vi "Write object configuration.vi"(4 "Present":bool=TRUE, 6 "Object name":string, 8 "Error In":errorcluster, 9 "Configuration":variant, 10 "File path":path, 11 "object":refnum<class>) -> (0 "Error Out":errorcluster, 1 "Section out":string, 2 "File path out":path)   [LabVIEW 2019]
uses:
  <vilib>/Utility/config.llb/NI_LVConfig.lvlib
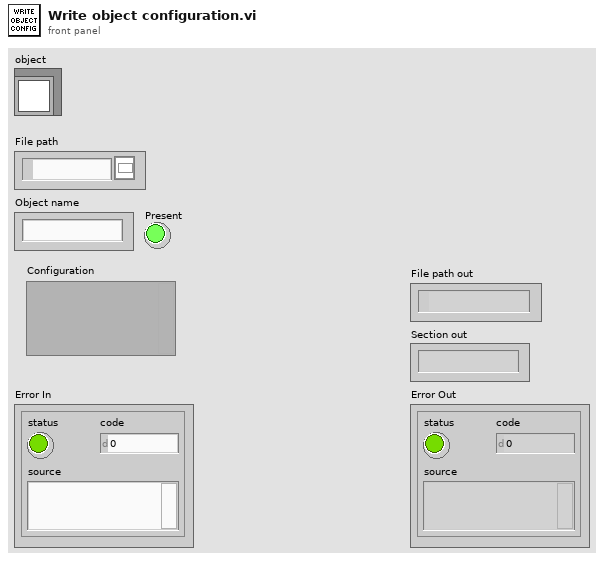
[diagram p1: front panel]
types:
  T1 = typedef "NI_LVConfig.lvlib/Config Data RefNum.ctl" = refnum<k1>
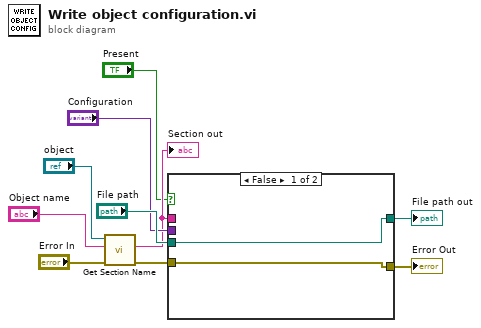
[diagram p0: block diagram]
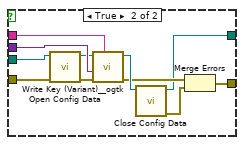
[diagram p2: hidden frame]
diagram:
  n1 = call "Get Section Name.vi"("Error In"="Error In", "Object name"="Object name", "object"="object") -> ("Error Out"=w3:errorcluster, "Section out"=w4:string)  [unwired: 7 in]
  "Section out" <- w4
  n2 = case shown="False" "Present" {
    tunnel: "File path" -> [w12 w23]
    tunnel: "Configuration" -> [_ w22]
    tunnel: [w12 w16] -> w8
    tunnel: [w11 w15] -> w7
    tunnel: w4 -> [_ w14]
    tunnel: w3 -> [w11 w13]
    frame False {
    }
    frame True {
      n3 = call <vilib>:"Open Config Data.vi"("error in (no error)"=w13, "configuration file path"=w23) -> ("error out"=w20:errorcluster, "refnum"=w21:T1)  [unwired: 7 in, 1 out]
      n4 = call <userlib>:"Write Key (Variant)__ogtk.vi"("section"=w14, "error in (no error)"=w20, "key-value"=w22, "refnum"=w21) -> ("error out"=w18:errorcluster, "refnum out"=w19:T1)  [unwired: 6 in]
      n5 = call <vilib>:"Close Config Data.vi"("refnum"=w19) -> ("error out"=w17:errorcluster, "file path"=w16:path)  [unwired: 9 in]
      n6 = Merge Errors(w18, w17) -> (w15:errorcluster)
    }
  }
  "File path out" <- w8
  "Error Out" <- w7
